vi "Fetch Waveform Measurement.vi"   [LabVIEW 2015, in "Tektronix 7000 Series.lvlib"]
doc: "Initiates a waveform acquisition on the specified channel(s) and returns a <B>Measurement</B> value. Use the Fetch Waveform Measurement VI separately for any other waveform measurement on a channel without initiating another acquisition."
uses:
  <instrlib>/Tektronix 7000 Series/Tektronix 7000 Series.lvlib
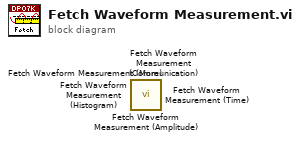
[diagram p0: block diagram]
diagram:
  n1 = call <instrlib>:"Fetch Waveform Measurement (Amplitude).vi"() -> ()  [unwired: 13 in, 3 out]
  n2 = call <instrlib>:"Fetch Waveform Measurement (Communication).vi"() -> ()  [unwired: 13 in, 3 out]
  n3 = call <instrlib>:"Fetch Waveform Measurement (Histogram).vi"() -> ()  [unwired: 13 in, 3 out]
  n4 = call <instrlib>:"Fetch Waveform Measurement (Time).vi"() -> ()  [unwired: 13 in, 3 out]
  n5 = call <instrlib>:"Fetch Waveform Measurement (More).vi"() -> ()  [unwired: 13 in, 3 out]
